vi "Globals HEWH.vi"() -> ()   [LabVIEW 2013]
panel:
  in  "Temperature Fault":u32(colorbox)=15698688
  in  "Bad Com Limit":i32=65
  in  "New Dryer Status String":string="New record"
  in  "Max Temp Alarm Limit":dbl=230.0
  in  "Fault Color":u32(colorbox)=16711680
  in  "Sub /R/N":string=" :: "
  in  "Save Data Array Length(56*11+1)":i32=617
  in  "Record Length for Sample Data":i32=11
  in  "Path: Data Backup":path=path "\\\\192.168.1.12\\share/Test Data/WILT"
  in  "Aisle Labels":string[](array[string])=["Aisle1", "Aisle1A", "Aisle2", "Aisle3", "Aisle4"]
  in  "History Header Data":string[](array[string])=["Completion Time", "Cum Time On", "Imax(L1)", "Imax(L2)", "Temp(max)"]
  in  "Sample Header Data":string[](array[string])=["Time", "Cycle Count", "Cum Time On", "ASCII", "Status", "I(L1)", "I(L2)", "Trmb", "V", "V2", "SW"]
  in  "UnConfigured":u32(colorbox)=7171459
  in  "Err Color":u32(colorbox)
  in  "Paused Color":u32(colorbox)=16860
  in  "Unknown Status Color":u32(colorbox)
  in  "Running Color":u32(colorbox)=6618880
  in  "Not Started Color":u32(colorbox)=16776960
  in  "Stopped Color":u32(colorbox)=16776960
  in  "No Com Color":u32(colorbox)
  in  "No Com Status Message":string="No Com"
  in  "Path: Save File":path=path "D:/data"
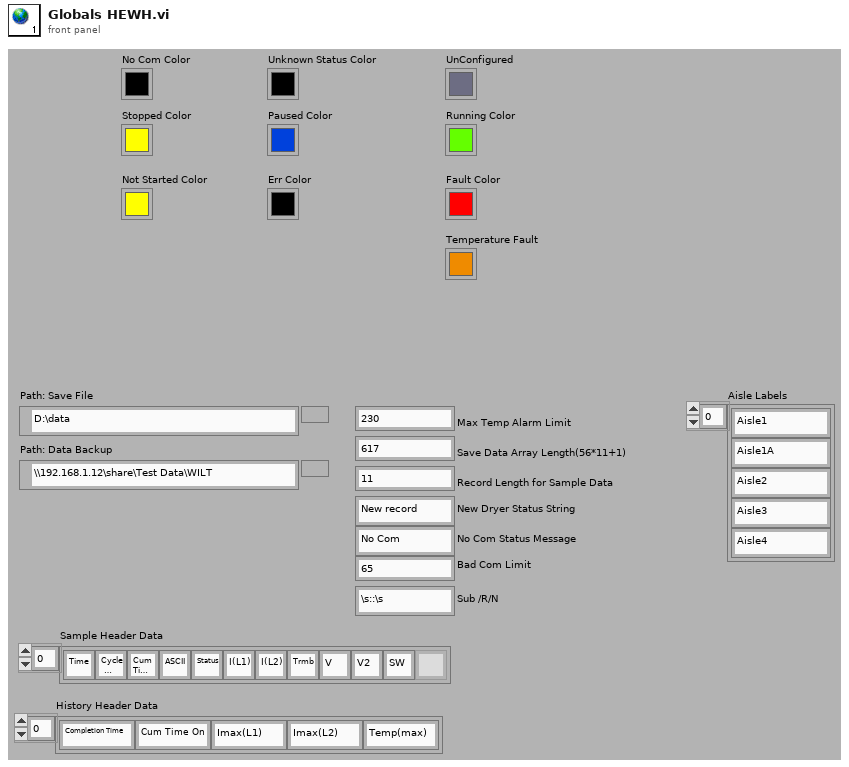
[diagram p1: front panel]
diagram:
